vi "ScaleBiasCluster.vi"(8 "Error In":errorcluster, 9 "Waveform in":waveform(dbl), 11 "ScaleBias":T1={"Scale"=100.0, "Bias"=100.0} {"Bias" format="%#_13g"; "Scale" format="%#_13g"}) -> (0 "Error Out":errorcluster, 3 "Waveform out":waveform(dbl))   [LabVIEW 2018]
uses:
  ScaleBias.ctl
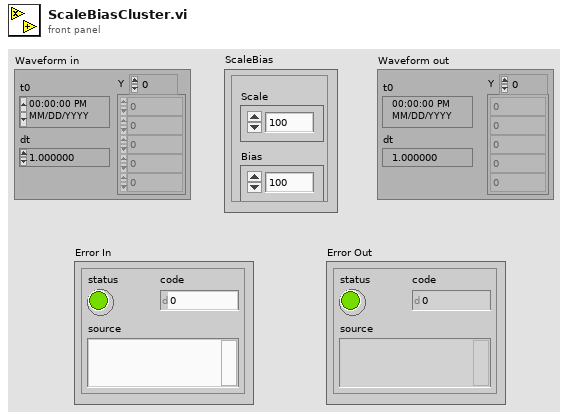
[diagram p1: front panel]
types:
  T1 = typedef "ScaleBias.ctl" = cluster{"Scale":dbl, "Bias":dbl}
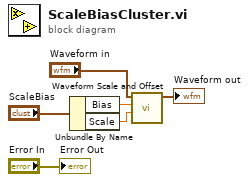
[diagram p0: block diagram]
diagram:
  n1 = Unbundle By Name("ScaleBias") -> ("Bias"=w3:dbl, "Scale"=w2:dbl)
  n2 = call <vilib>:"Waveform Scale and Offset.vi"("scale"=w2, "offset"=w3, "waveform in"="Waveform in") -> ("waveform out"=→"Waveform out":waveform(dbl))  [unwired: 7 in, 1 out]
  "Error Out" <- "Error In"
